vi "calculate last byte.vi"(9 "Input Length":u8, 10 "type":T1, 11 "byte in":i32) -> (3 "last byte":i32)   [LabVIEW 2013, in "Profibus Module runtime.lvclass"]
uses:
  Profibus Module runtime.lvclass
  <vilib>/NI/Tag Bus/tag/Data Type.ctl
  <vilib>/NI/Tag Bus/tag/tag descriptor.lvclass
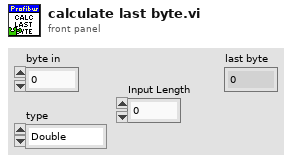
[diagram p1: front panel]
types:
  T1 = typedef "tag bus.lvlib/tag descriptor.lvclass/Data Type.ctl" = enum16{"Double", "Single", "I64", "I32", "I16", "I8", "U64", "U32", "U16", "U8", "Boolean", "String", "Array of Double", "Array of Single", "Array of I64", "Array of I32", "Array of I16", "Array of I8", "Array of U64", "Array of U32", "Array of U16", "Array of U8", "Array of Boolean", "Array of String"}
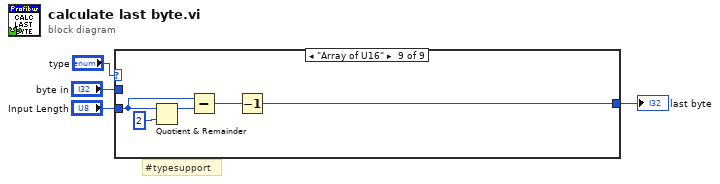
[diagram p0: block diagram]
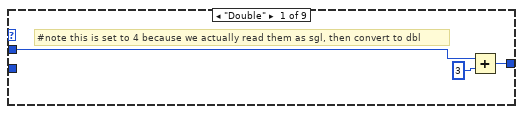
[diagram p2: hidden frame]
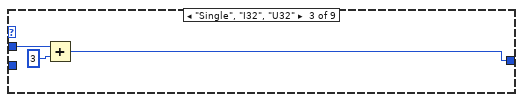
[diagram p4: hidden frame]
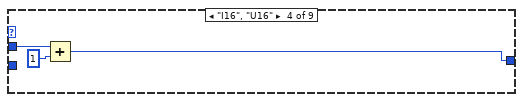
[diagram p5: hidden frame]
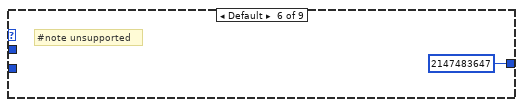
[diagram p7: hidden frame]
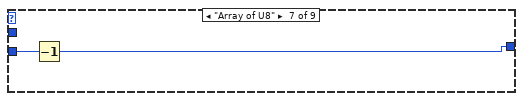
[diagram p8: hidden frame]
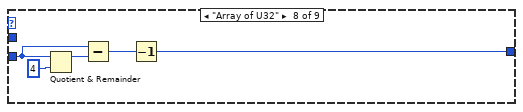
[diagram p9: hidden frame]
diagram:
  # "#typesupport"
  n1 = case shown="\"Array of U16\"" "type" {
    tunnel: "byte in" -> [w5 w8 w11 w14 w15 _ _ _ _]
    tunnel: [w6 w8 w9 w12 w15 2147483647 ("byte in") w17 w19 w24] -> w2
    tunnel: "Input Length" -> [_ _ _ _ _ _ w18 w22 w27]
    frame "Double" {
      # "#note this is set to 4 because we actually read them as sgl, then convert to dbl"
      n2 = Add(x=w5, y=3) -> (x+y=w6:i32)
    }
    frame "Boolean" {
    }
    frame "Single", "I32", "U32" {
      n3 = Add(x=w11, y=3) -> (x+y=w9:i32)
    }
    frame "I16", "U16" {
      n4 = Add(x=w14, y=1) -> (x+y=w12:i32)
    }
    frame "I8", "U8" {
    }
    frame Default {
      # "#note unsupported"
    }
    frame "Array of U8" {
      n5 = Decrement(x=w18) -> (x-1=w17:u8)
    }
    frame "Array of U32" {
      n6 = Quotient & Remainder(x=w22, y=u8 4) -> (x-y*floor(x/y)=w21:u8)  [unwired: 1 out]
      n7 = Subtract(x=w22, y=w21) -> (x-y=w20:u8)
      n8 = Decrement(x=w20) -> (x-1=w19:u8)
    }
    frame "Array of U16" {
      n9 = Quotient & Remainder(x=w27, y=u8 2) -> (x-y*floor(x/y)=w26:u8)  [unwired: 1 out]
      n10 = Subtract(x=w27, y=w26) -> (x-y=w25:u8)
      n11 = Decrement(x=w25) -> (x-1=w24:u8)
    }
  }
  "last byte" <- w2
